vi "Test harness - Is part of the LabVIEW install folder.vi"(11 "Type of file to test":T1=".vi") -> (0 "error out":errorcluster, 3 "Library member part of vi.lib":bool)   [LabVIEW 2021]
uses:
  Test harness file type.ctl
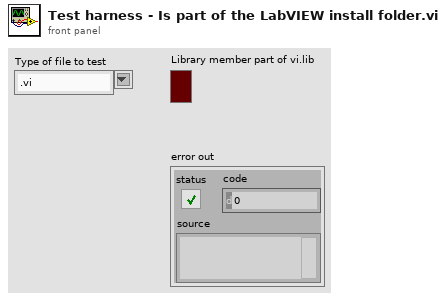
[diagram p1: front panel]
types:
  T1 = typedef "Test harness file type.ctl" = string
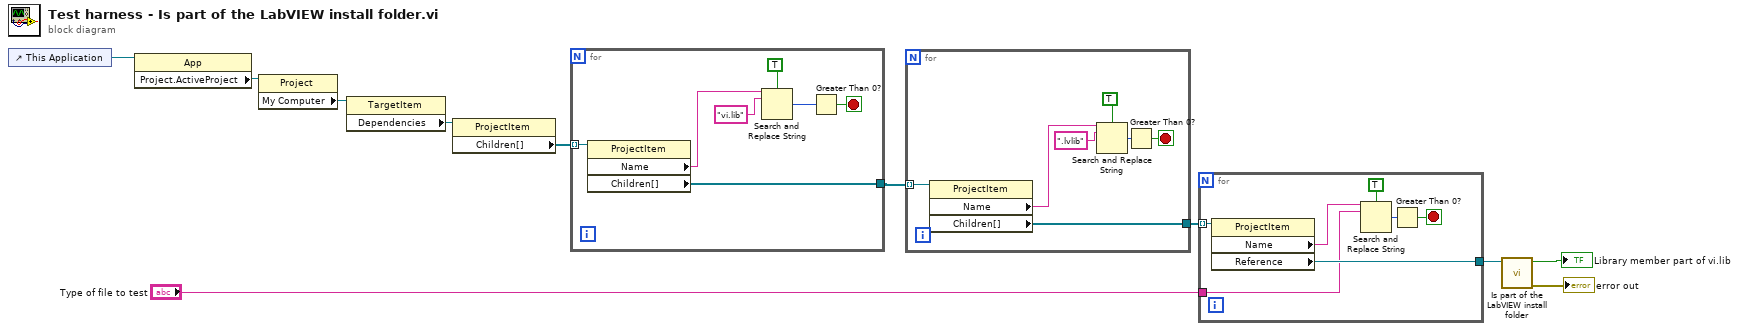
[diagram p0: block diagram]
diagram:
  n1 = control-ref of="This Application"() -> (w2:refnum<vi>)
  n2 = property class="App"(reference=w2) -> ("Project.ActiveProject"=w11:refnum<vi>)  [unwired: 1 in, 2 out]
  n3 = property class="Project"(reference=w11) -> ("My Computer"=w8:refnum<vi>)  [unwired: 1 in, 2 out]
  n4 = property class="TargetItem"(reference=w8) -> ("Dependencies"=w10:refnum<vi>)  [unwired: 1 in, 2 out]
  n5 = property class="ProjectItem"(reference=w10) -> ("Children[]"=w9:refnum<vi>[])  [unwired: 1 in, 2 out]
  n6 = for {
    tunnel: w9 -> [w18] mode=indexing
    tunnel: [w13] -> w7
    stop <- w17 stop-if-true
    n7 = property class="ProjectItem"(reference=w18) -> ("Name"=w16:string, "Children[]"=w13:refnum<vi>[])  [unwired: 1 in, 2 out]
    n8 = Search and Replace String(case sensitive?=TRUE ("ignore case? (F)"), input string=w16, search string="vi.lib" ("search string/char (-)")) -> (number of replacements=w12:i32)  [unwired: 5 in, 3 out]
    n9 = Greater Than 0?(x=w12) -> (x > 0?=w17:bool)
  }
  n10 = for {
    tunnel: w7 -> [w25] mode=indexing
    tunnel: [w20] -> w6
    stop <- w21 stop-if-true
    n11 = property class="ProjectItem"(reference=w25) -> ("Name"=w22:string, "Children[]"=w20:refnum<vi>[])  [unwired: 1 in, 2 out]
    n12 = Search and Replace String(case sensitive?=TRUE ("ignore case? (F)"), input string=w22, search string=".lvlib" ("search string/char (-)")) -> (number of replacements=w19:i32)  [unwired: 5 in, 3 out]
    n13 = Greater Than 0?(x=w19) -> (x > 0?=w21:bool)
  }
  n14 = for {
    tunnel: w6 -> [w32] mode=indexing
    tunnel: [w28] -> w4
    tunnel: "Type of file to test" -> [w26]
    stop <- w29 stop-if-true
    n15 = property class="ProjectItem"(reference=w32) -> ("Name"=w30:string, "Reference"=w28:refnum<vi>)  [unwired: 1 in, 2 out]
    n16 = Search and Replace String(case sensitive?=TRUE ("ignore case? (F)"), input string=w30, search string=w26) -> (number of replacements=w27:i32)  [unwired: 5 in, 3 out]
    n17 = Greater Than 0?(x=w27) -> (x > 0?=w29:bool)
  }
  n18 = call "Is part of the LabVIEW install folder.vi"("VI Reference"=w4) -> ("error out"=→"error out":errorcluster, "Is part of LabVIEW install folder"=→"Library member part of vi.lib":bool)  [unwired: 9 in]
